vi "Create (Single).vi"(10 "error in (no error)":errorcluster, 11 "Binding":string) -> (2 "error out":errorcluster, 3 "IP Resolver":refnum<class "IP Resolver.lvclass">)   [LabVIEW 2020, in "Vecto.lvlib" / "IP Resolver.lvclass"]
uses:
  IP Resolver.lvclass
  IP Resolver.lvclass/IP Resolver.ctl
  Address Type.ctl
  Bind Info.ctl
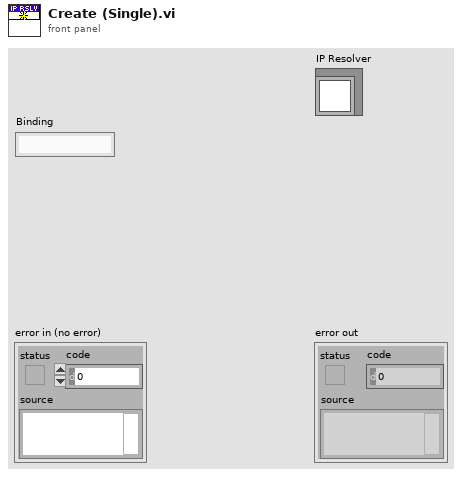
[diagram p1: front panel]
types:
  T1 = typedef "Vecto.lvlib/IP Resolver.lvclass/Address Type.ctl" = enum16{"Unknown", "Specific", "Subnet", "Any"}
  T2 = typedef "Vecto.lvlib/IP Resolver.lvclass/Bind Info.ctl" = cluster{"Type":T1, "Binding":string, "Subnet Bits":i32}
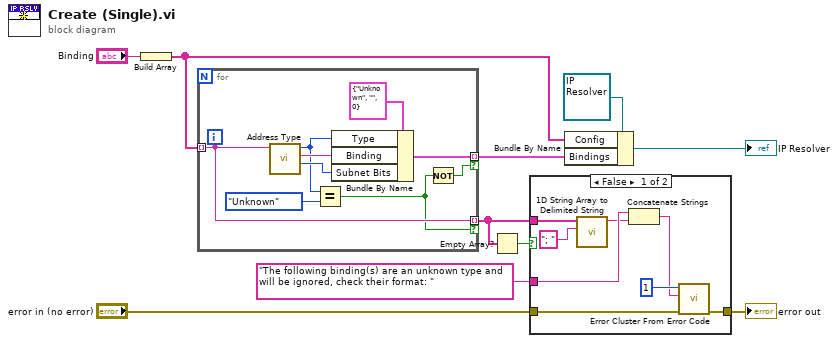
[diagram p0: block diagram]
diagram:
  n1 = Build Array("Binding") -> (w1:string[])
  n2 = for {
    tunnel: w1 -> [w12] mode=indexing
    tunnel: [w16] -> w8 mode=indexing if=w13
    tunnel: [w12] -> w6 mode=indexing if=w11
    n3 = call "Address Type.vi"("Address In"=w12) -> ("Subnet Bits"=w17:i32, "Address"=w18:string, "Address Type"=w15:T1)  [unwired: 8 in]
    n4 = Equal?(x=w15, y=Address_Type."Unknown") -> (x = y?=w11:bool)
    n5 = Bundle By Name(cluster=T2 {"Type"=enum."Unknown", "Binding"="", "Subnet Bits"=0} ("Bind Info"), "Type"=w15, "Binding"=w18, "Subnet Bits"=w17) -> (w16:T2)
    n6 = Not(x=w11) -> (.not. x?=w13:bool)
  }
  n7 = Empty Array?(array=w6) -> (empty?=w5:bool)
  n8 = case shown="False" w5 {
    tunnel: w6 -> [w27 _]
    tunnel: "error in (no error)" -> [w23 w28]
    tunnel: [w20 w28] -> w3
    tunnel: "The following binding(s) are an unknown type and will be ignored, check their format: " -> [w25 _]
    frame False {
      n9 = call <vilib>:"1D String Array to Delimited String.vi"("delimiter"="; ", "string array"=w27) -> ("delimited string"=w24:string)  [unwired: 9 in]
      n10 = Concatenate Strings(w25, w24) -> (w21:string)
      n11 = call <vilib>:"Error Cluster From Error Code.vi"("error in (no error)"=w23, "error message (\"\")"=w21, "error code (0)"=1) -> ("error out"=w20:errorcluster)  [unwired: 6 in]
    }
    frame True {
    }
  }
  "error out" <- w3
  n12 = Bundle By Name(cluster=refnum<class "IP Resolver.lvclass"> refnum ("IP Resolver in"), "Config"=w1, "Bindings"=w8) -> (→"IP Resolver":refnum<class "IP Resolver.lvclass">)
